vi "Facade.vi"(0 "Data In":T7={"Slider"={"Numeric"=25.0, "Numeric"=0.0, "Numeric"=0.0}, "Digital display"=0.0, "end_timer"=TRUE} {"Slider" scale=0.0..500.0 scale format="%#_5g"}, 2 "Display State In":T3={"SP_Source"={"connect"=FALSE, "SP_Source"=enum."initialize", "SP_Set"=0.0, "SP"=0.0}, "Write"=FALSE, "button state"=enum."init", "reset_timer"=FALSE, "load_timer"=FALSE, "Time"=0, "t ms"=0, "tick"=0, "scale maximum"=100.0}, 3 "Container State":T6) -> (6 "Data Out":T7={"Slider"={"Numeric"=25.0, "Numeric"=0.0, "Numeric"=0.0}, "Digital display"=0.0, "end_timer"=TRUE} {"Slider" scale=0.0..500.0 scale format="%#_5g"}, 7 "Display State Out":T3={"SP_Source"={"connect"=FALSE, "SP_Source"=enum."initialize", "SP_Set"=0.0, "SP"=0.0}, "Write"=FALSE, "button state"=enum."init", "reset_timer"=FALSE, "load_timer"=FALSE, "Time"=0, "t ms"=0, "tick"=0, "scale maximum"=100.0}, 8 "Action":T2)   [LabVIEW 2019, in "control.lvlib" / "SP_h1.xctl"]
uses:
  SP_h1.xctl
  Data.ctl
  <vilib>/_xctls/Container State.ctl
  State.ctl
  Heating/ctl/Y_source.ctl
  Y_controlState.ctl
  <vilib>/_xctls/Action.ctl
  <vilib>/_xctls/XControlSupport.lvlib
  Timer Delay/Timers.lvlib
  Heating/Heating.lvlib
panel:
  in  "setpoint":dbl step=1.0 format="%#.1f"
  in  "slider":T1(slide) scale=0.0..1000.0 scale format="%#.0f"
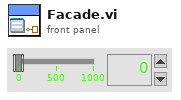
[diagram p1: front panel]
types:
  T1 = cluster{"Numeric":dbl, "Numeric":dbl, "Numeric":dbl}
  T2 = typedef "XControlSupport.lvlib/Action.ctl" = cluster{"Data Changed?":bool, "State Changed?":bool, "Action Name":string}
  T3 = typedef "control.lvlib/SP_h1.xctl/State.ctl" = cluster{"SP_Source":cluster{"connect":bool, "SP_Source":T4, "SP_Set":dbl, "SP":dbl}, "Write":bool, "button state":T5, "reset_timer":bool, "load_timer":bool, "Time":u32, "t ms":u32, "tick":u32, "scale maximum":dbl}
  T4 = typedef "Heating.lvlib/Y_source.ctl" = enum8{"initialize", "local disabled", "local hand", "hand", "auto", "dist"}
  T5 = typedef "control.lvlib/SP_h1.xctl/Y_controlState.ctl" = enum16{"init", "not connect", "local disabled", "local hand", "hand", "value change", "auto", "dist"}
  T6 = typedef "XControlSupport.lvlib/Container State.ctl" = cluster{"Indicator?":bool, "Run Mode?":bool, " Refnum":refnum<vi>}
  T7 = typedef "control.lvlib/SP_h1.xctl/Data.ctl" = cluster{"Slider":cluster{"Numeric":dbl, "Numeric":dbl, "Numeric":dbl}, "Digital display":dbl, "end_timer":bool}
  T8 = enum8{"Enabled", "Disabled", "Disabled and Grayed Out"}
  T9 = cluster{"Numeric":dbl, "NewVal":dbl, "Numeric":dbl}
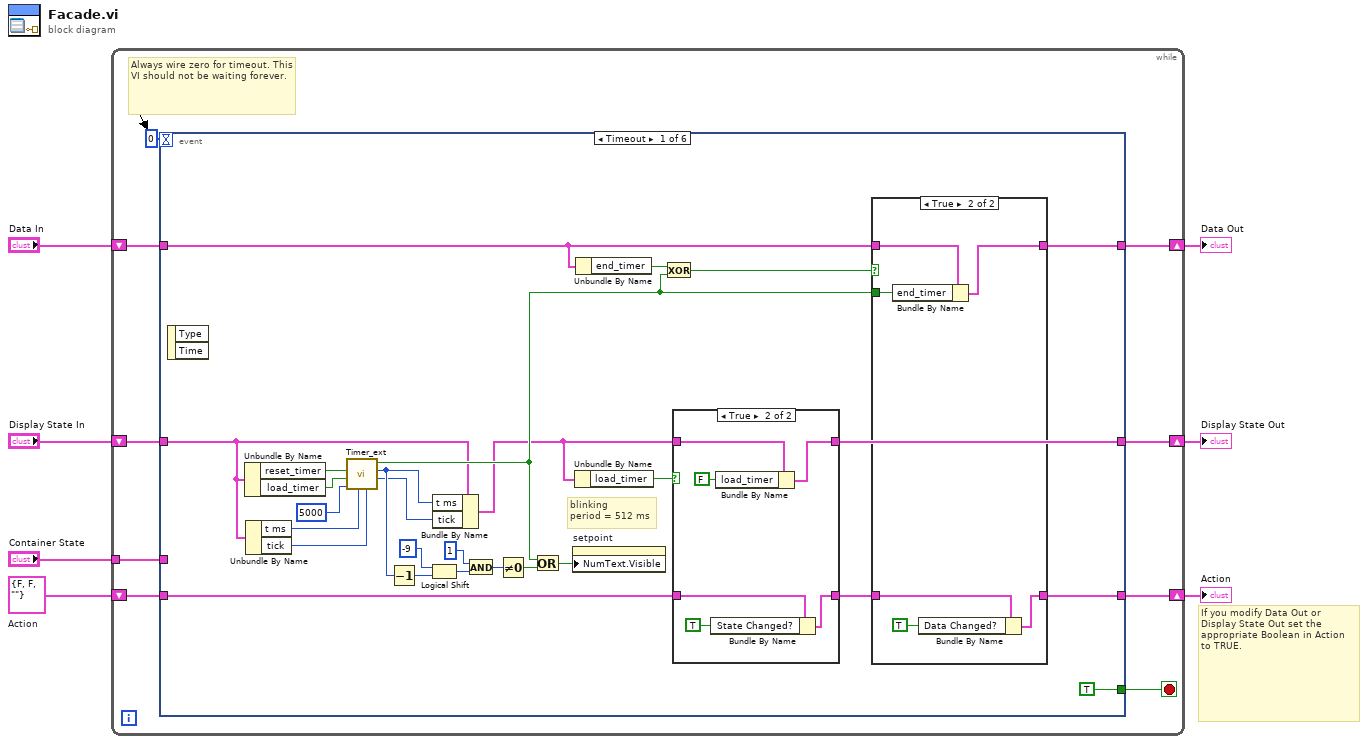
[diagram p0: block diagram]
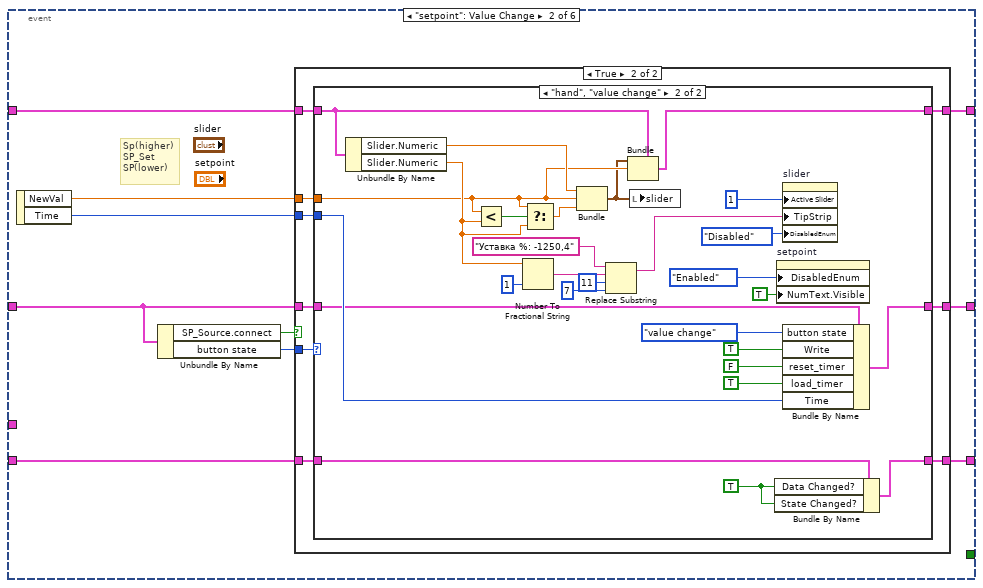
[diagram p4: hidden frame]
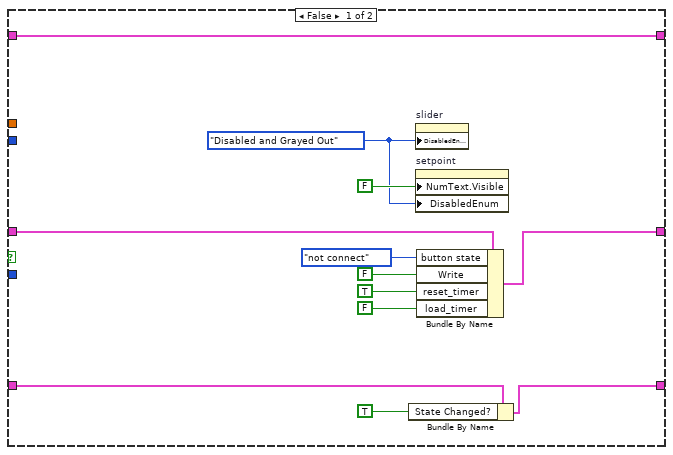
[diagram p5: hidden frame]
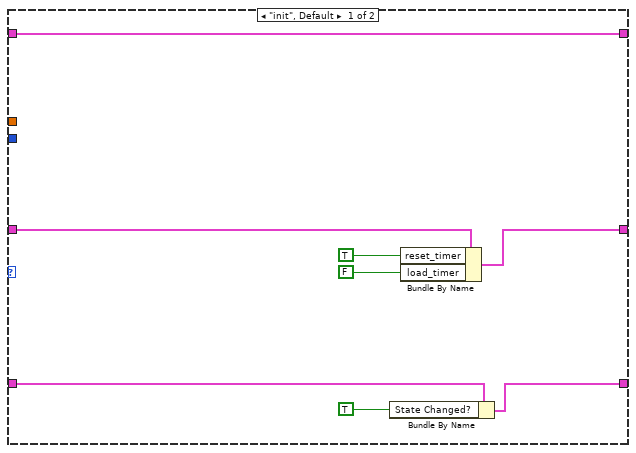
[diagram p6: hidden frame]
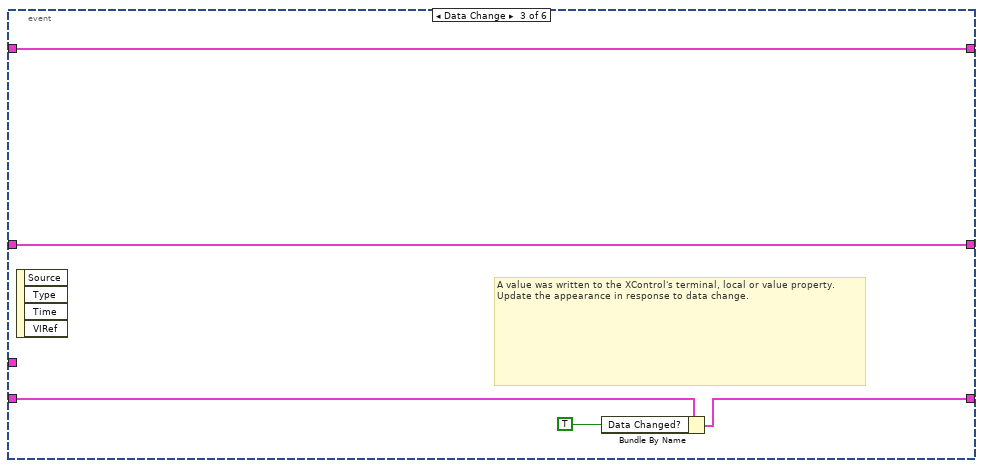
[diagram p7: hidden frame]
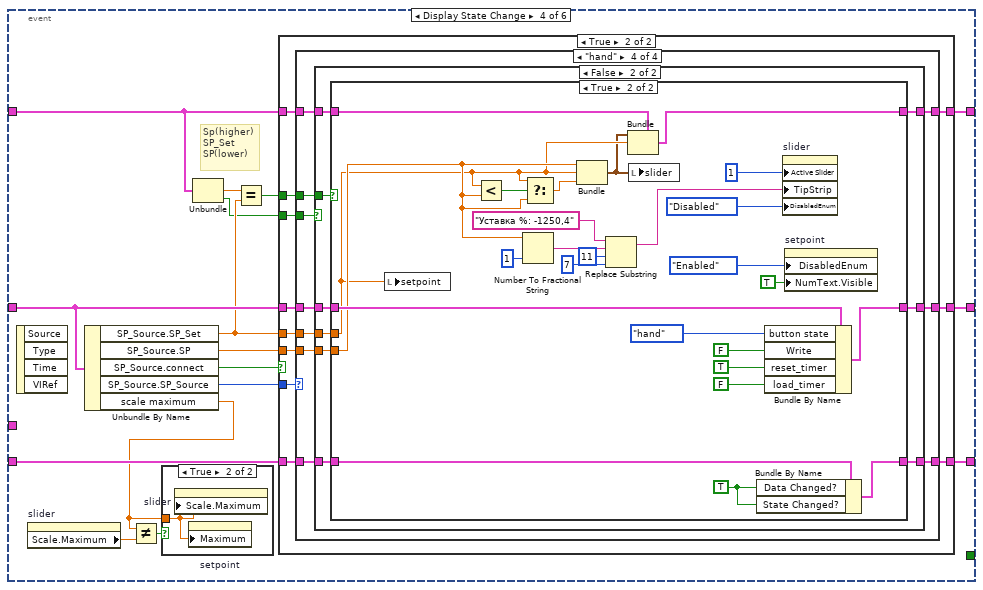
[diagram p8: hidden frame]
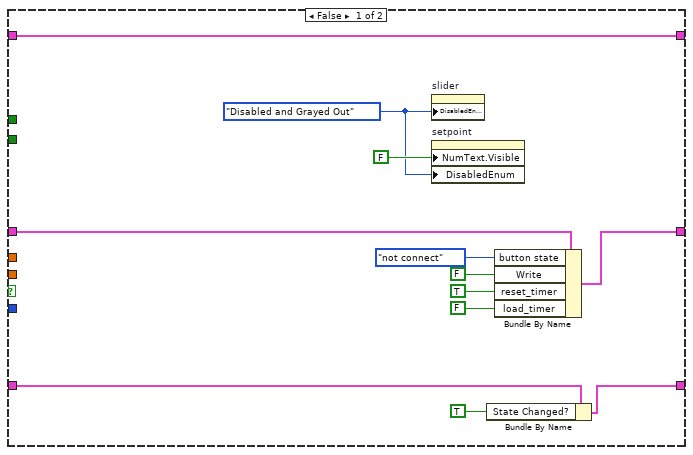
[diagram p10: hidden frame]
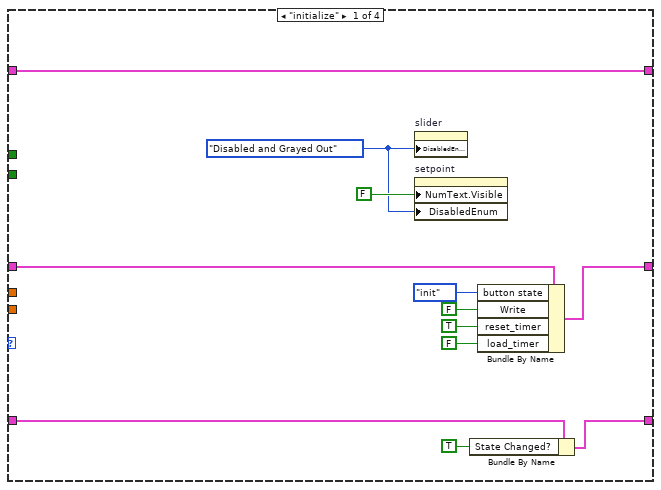
[diagram p11: hidden frame]
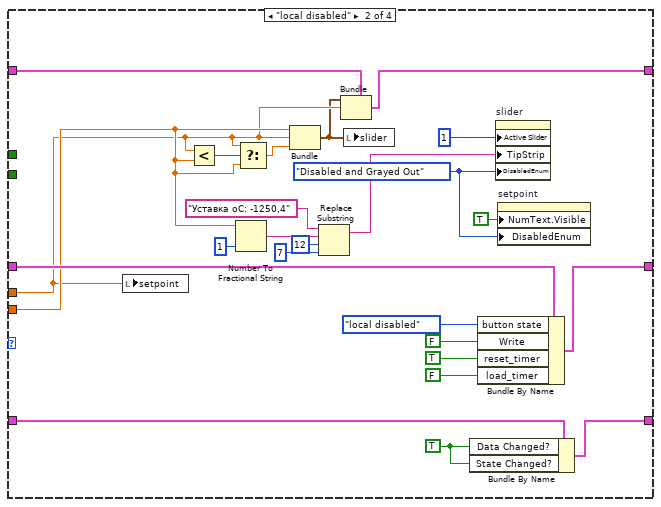
[diagram p12: hidden frame]
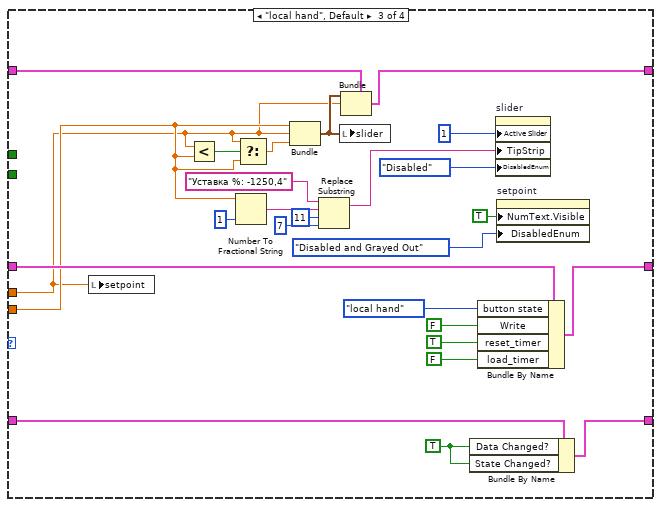
[diagram p13: hidden frame]
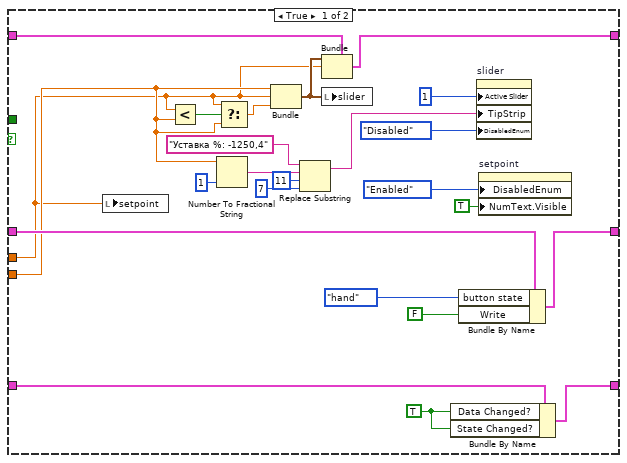
[diagram p14: hidden frame]
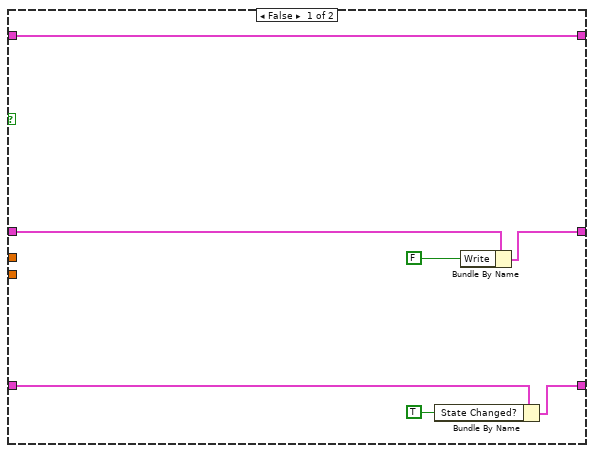
[diagram p15: hidden frame]
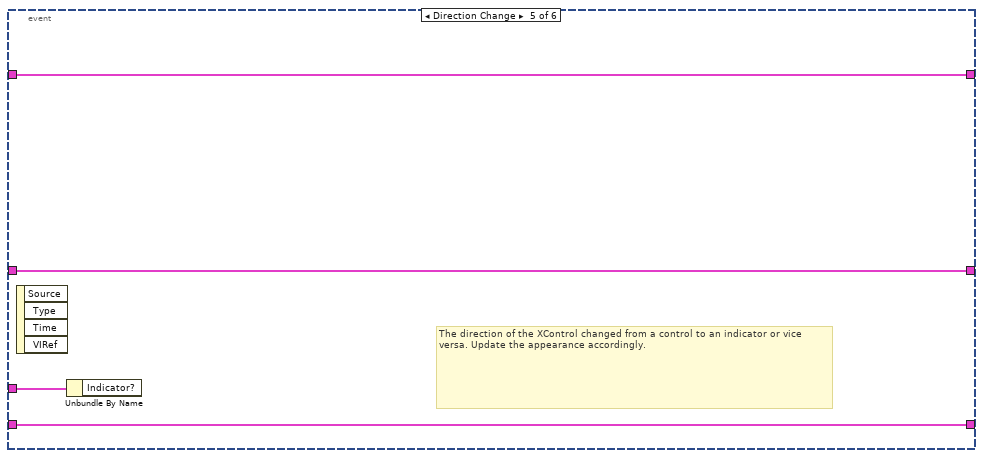
[diagram p16: hidden frame]
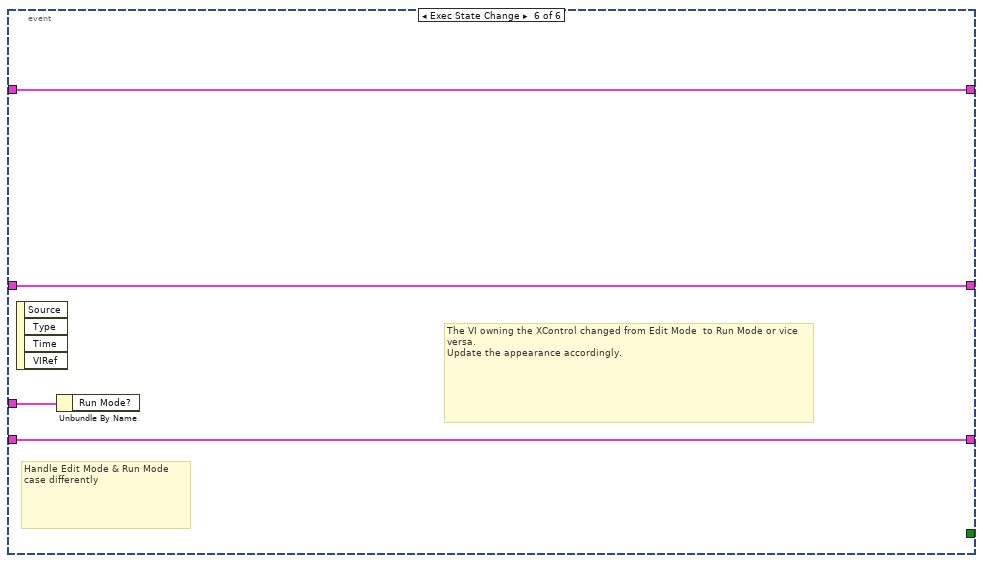
[diagram p17: hidden frame]
diagram:
  w1 = T2 {"Data Changed?"=FALSE, "State Changed?"=FALSE, "Action Name"=""}  # Action
  # "If you modify Data Out or\nDisplay State Out set the\nappropriate Boolean in Action\nto TRUE."
  n1 = while {
    shift-right: [w9] -> w4
    shift-left: "Display State In" -> [w16]
    tunnel: "Container State" -> [w13]
    shift-right: [w8] -> w7
    shift-left: "Data In" -> [w12]
    shift-right: [w10] -> w2
    shift-left: w1 -> [w11]
    stop <- w15 stop-if-true
    # "Always wire zero for timeout. This\nVI should not be waiting forever."
    n2 = event shown="[0] Timeout" {
      selector: _ -> [_ _ _ _ _ _]
      dyn-events: _ -> [_ _ _ _ _ _]
      timeout: 0 -> [_ _ _ _ _ _]
      tunnel: w16 -> [w17 w64 w130 w142 w313 w317]
      tunnel: [w40 w69 w130 w146 w313 w317] -> w9
      tunnel: [TRUE _ _ _ _ _] -> w15
      tunnel: w13 -> [_ _ _ _ w314 w318]
      tunnel: w12 -> [w28 w68 w131 w138 w312 w316]
      tunnel: [w31 w67 w131 w147 w312 w316] -> w8
      tunnel: [w23 w65 w128 w144 w311 w315] -> w10
      tunnel: w11 -> [w29 w66 w127 w145 w311 w315]
      event Timeout {
        # "blinking\nperiod = 512 ms"
        n3 = event-data() -> ()  [unwired: 1 in, 2 out]
        n4 = Unbundle By Name(w17) -> ("reset_timer"=w42:bool, "load_timer"=w41:bool)
        n5 = Unbundle By Name(w17) -> ("t ms"=w22:u32, "tick"=w21:u32)
        n6 = call "Timer_ext.vi"("tick old"=w21, "t ms old"=w22, "ms"=u32 5000, "Load"=w41, "Reset"=w42) -> ("tick"=w19:u32, "t ms"=w20:u32, "End"=w26:bool)  [unwired: 4 in]
        n7 = Decrement(x=w20) -> (x-1=w37:u32)
        n8 = Logical Shift(y=i16 -9, x=w37) -> (x << y=w35:u32)
        n9 = Bundle By Name(cluster=w17, "t ms"=w20, "tick"=w19) -> (w18:T3)
        n10 = And(x=u32 1 ("y"), y=w35) -> (x .and. y?=w33:u32)
        n11 = Not Equal To 0?(x=w33) -> (x != 0?=w38:bool)
        n12 = Or(x=w26, y=w38) -> (x .or. y?=w32:bool)
        n13 = property on="setpoint" class="DigNum (strict)"("NumText.Visible"=w32) -> ()  [unwired: 2 in, 2 out]
        n14 = Unbundle By Name(w18) -> ("load_timer"=w30:bool)
        n15 = Unbundle By Name(w28) -> ("end_timer"=w27:bool)
        n16 = Exclusive Or(1:w26, 2:w27) -> (0:w25:bool)
        n17 = case shown="True" w30 {
          tunnel: [w53 w59] -> w40
          tunnel: w18 -> [w53 w57]
          tunnel: w29 -> [w52 w55]
          tunnel: [w52 w54] -> w24
          frame False {
          }
          frame True {
            n18 = Bundle By Name(cluster=w55, "State Changed?"=TRUE ("Data Changed?")) -> (w54:T2)
            n19 = Bundle By Name(cluster=w57, "load_timer"=FALSE) -> (w59:T3)
          }
        }
        n20 = case shown="True" w25 {
          tunnel: [w44 w51] -> w31
          tunnel: w28 -> [w44 w50]
          tunnel: w26 -> [_ w49]
          tunnel: w24 -> [w45 w47]
          tunnel: [w45 w46] -> w23
          frame False {
          }
          frame True {
            n21 = Bundle By Name(cluster=w50, "end_timer"=w49) -> (w51:T7)
            n22 = Bundle By Name(cluster=w47, "Data Changed?"=TRUE) -> (w46:T2)
          }
        }
      }
      event "setpoint": Value Change {
        # "Sp(higher)\nSP_Set\nSP(lower)"
        n23 = event-data() -> ("NewVal"=w61:dbl, "Time"=w60:u32)  [unwired: 1 in]
        n24 = Unbundle By Name(w64) -> ("SP_Source.connect"=w63:bool, "button state"=w62:T5)
        n25 = case shown="True" w63 {
          tunnel: w62 -> [_ w90]
          tunnel: w64 -> [w80 w89]
          tunnel: [w79 w88] -> w69
          tunnel: w68 -> [w72 w87]
          tunnel: [w72 w86] -> w67
          tunnel: w66 -> [w77 w84]
          tunnel: [w76 w85] -> w65
          tunnel: w61 -> [_ w83]
          tunnel: w60 -> [_ w82]
          frame False {
            w70 = T8."Disabled and Grayed Out" ("Disabled")
            n26 = Bundle By Name(cluster=w77, "State Changed?"=TRUE ("Data Changed?")) -> (w76:T2)
            n27 = property on="slider" class="Slide (strict)"("DisabledEnum"=w70) -> ()  [unwired: 2 in, 2 out]
            n28 = property on="setpoint" class="DigNum (strict)"("NumText.Visible"=FALSE ("Z_ASwitch"), "DisabledEnum"=w70) -> ()  [unwired: 2 in, 2 out]
            n29 = Bundle By Name(cluster=w80, "button state"=Y_controlState."not connect" ("f 3"), "Write"=FALSE ("Z_ASwitch"), "reset_timer"=TRUE ("Z_ASwitch"), "load_timer"=FALSE ("Z_ASwitch")) -> (w79:T3)
          }
          frame True {
            n30 = case shown="\"hand\", \"value change\"" w90 {
              tunnel: w89 -> [w97 w108]
              tunnel: [w96 w126] -> w88
              tunnel: w87 -> [w91 w105]
              tunnel: [w91 w107] -> w86
              tunnel: [w93 w124] -> w85
              tunnel: w84 -> [w94 w125]
              tunnel: w83 -> [_ w102]
              tunnel: w82 -> [_ w109]
              frame "init", Default {
                # "local hand"
                n31 = Bundle By Name(cluster=w94, "State Changed?"=TRUE ("Data Changed?")) -> (w93:T2)
                n32 = Bundle By Name(cluster=w97, "reset_timer"=TRUE, "load_timer"=FALSE) -> (w96:T3)
              }
              frame "hand", "value change" {
                w120 = TRUE ("Data Changed?")
                # "local hand"
                n33 = Unbundle By Name(w105) -> ("Slider.Numeric"=w104:dbl, "Slider.Numeric"=w103:dbl)
                n34 = Less?(x=w102, y=w103) -> (x < y?=w113:bool)
                n35 = Number To Fractional String(number=w103, precision (6)=i16 1) -> (F-format string=w116:string)  [unwired: 2 in]
                n36 = Select(t=w102, s=w113, f=w103) -> (s? t:f=w112:dbl)
                n37 = Bundle("Numeric"=w104, "NewVal"=w102, "Numeric"=w112) -> (w99:T9)  [unwired: 1 in]
                n38 = Replace Substring(2:7 ("length (len. of substring)"), 3:11 ("offset (0)"), 4:w116, 5:"Уставка %: -1250,4") -> (1:w110:string)  [unwired: 1 out]
                n39 = Bundle(cluster=w105, "Slider"=w99, "Digital display"=w102) -> (w107:T7)  [unwired: 1 in]
                n40 = local write "slider"(w99) -> ()
                n41 = Bundle By Name(cluster=w125, "Data Changed?"=w120, "State Changed?"=w120) -> (w124:T2)
                n42 = property on="setpoint" class="DigNum (strict)"("DisabledEnum"=T8."Enabled" ("Disabled"), "NumText.Visible"=TRUE ("Numeric Text.Visible")) -> ()  [unwired: 2 in, 2 out]
                n43 = property on="slider" class="Slide (strict)"("Active Slider"=1, "TipStrip"=w110, "DisabledEnum"=T8."Disabled" ("Disabled")) -> ()  [unwired: 2 in, 2 out]
                n44 = Bundle By Name(cluster=w108, "button state"=Y_controlState."value change" ("f 3"), "Write"=TRUE ("Z_ASwitch"), "reset_timer"=FALSE ("Z_ASwitch"), "load_timer"=TRUE ("Z_ASwitch"), "Time"=w109) -> (w126:T3)
              }
            }
          }
        }
      }
      event Data Change {
        # "A value was written to the XControl's terminal, local or value property.\nUpdate the appearance in response to data change."
        n45 = event-data() -> ()  [unwired: 1 in, 4 out]
        n46 = Bundle By Name(cluster=w127, "Data Changed?"=TRUE) -> (w128:T2)
      }
      event Display State Change {
        # "Sp(higher)\nSP_Set\nSP(lower)"
        n47 = event-data() -> ()  [unwired: 1 in, 4 out]
        n48 = property on="slider" class="Slide (strict)"() -> ("Scale.Maximum"=w135:dbl)  [unwired: 2 in, 2 out]
        n49 = Unbundle By Name(w142) -> ("SP_Source.SP_Set"=w136:dbl, "SP_Source.SP"=w139:dbl, "SP_Source.connect"=w143:bool, "SP_Source.SP_Source"=w141:T4, "scale maximum"=w134:dbl)
        n50 = Not Equal?(x=w134, y=w135) -> (x != y?=w133:bool)
        n51 = case shown="True" w133 {
          tunnel: w134 -> [_ w148]
          frame False {
          }
          frame True {
            n52 = property on="slider" class="Slide (strict)"("Scale.Maximum"=w148) -> ()  [unwired: 2 in, 2 out]
            n53 = property on="setpoint" class="DigNum (strict)"("Maximum"=w148) -> ()  [unwired: 2 in, 2 out]
          }
        }
        n54 = Unbundle(w138) -> ("Digital display"=w137:dbl, "end_timer"=w132:bool)  [unwired: 1 out]
        n55 = Equal?(x=w137, y=w136) -> (x = y?=w140:bool)
        n56 = case shown="True" w143 {
          tunnel: w141 -> [_ w171]
          tunnel: w142 -> [w159 w170]
          tunnel: [w158 w169] -> w146
          tunnel: w138 -> [w151 w168]
          tunnel: [w151 w167] -> w147
          tunnel: w145 -> [w156 w165]
          tunnel: [w155 w166] -> w144
          tunnel: w132 -> [_ w164]
          tunnel: w139 -> [_ w163]
          tunnel: w140 -> [_ w162]
          tunnel: w136 -> [_ w161]
          frame False {
            w149 = T8."Disabled and Grayed Out" ("Disabled")
            n57 = property on="slider" class="Slide (strict)"("DisabledEnum"=w149) -> ()  [unwired: 2 in, 2 out]
            n58 = property on="setpoint" class="DigNum (strict)"("NumText.Visible"=FALSE ("Z_ASwitch"), "DisabledEnum"=w149) -> ()  [unwired: 2 in, 2 out]
            n59 = Bundle By Name(cluster=w156, "State Changed?"=TRUE ("Data Changed?")) -> (w155:T2)
            n60 = Bundle By Name(cluster=w159, "button state"=Y_controlState."not connect" ("f 3"), "Write"=FALSE ("Z_ASwitch"), "reset_timer"=TRUE ("Z_ASwitch"), "load_timer"=FALSE ("Z_ASwitch")) -> (w158:T3)
          }
          frame True {
            n61 = case shown="\"hand\"" w171 {
              tunnel: w170 -> [w183 w208 w234 w244]
              tunnel: [w182 w207 w233 w243] -> w169
              tunnel: w168 -> [w174 w189 w214 w237]
              tunnel: [w174 w190 w215 w238] -> w167
              tunnel: [w180 w205 w231 w241] -> w166
              tunnel: w165 -> [w181 w206 w232 w242]
              tunnel: w164 -> [_ _ _ w240]
              tunnel: w163 -> [_ w188 w212 w239]
              tunnel: w162 -> [_ _ _ w236]
              tunnel: w161 -> [_ w185 w209 w235]
              frame "initialize" {
                w172 = T8."Disabled and Grayed Out" ("Disabled")
                # "local hand"
                n62 = property on="slider" class="Slide (strict)"("DisabledEnum"=w172) -> ()  [unwired: 2 in, 2 out]
                n63 = property on="setpoint" class="DigNum (strict)"("NumText.Visible"=FALSE ("Z_ASwitch"), "DisabledEnum"=w172) -> ()  [unwired: 2 in, 2 out]
                n64 = Bundle By Name(cluster=w181, "State Changed?"=TRUE ("Data Changed?")) -> (w180:T2)
                n65 = Bundle By Name(cluster=w183, "button state"=Y_controlState."init" ("f 3"), "Write"=FALSE ("Z_ASwitch"), "reset_timer"=TRUE ("Z_ASwitch"), "load_timer"=FALSE ("Z_ASwitch")) -> (w182:T3)
              }
              frame "local disabled" {
                w186 = T8."Disabled and Grayed Out" ("Disabled")
                w200 = TRUE ("Data Changed?")
                # "local hand"
                n66 = local write "setpoint"(w185) -> ()
                n67 = Less?(x=w185, y=w188) -> (x < y?=w194:bool)
                n68 = Number To Fractional String(number=w188, precision (6)=i16 1) -> (F-format string=w197:string)  [unwired: 2 in]
                n69 = Select(t=w185, s=w194, f=w188) -> (s? t:f=w193:dbl)
                n70 = Bundle("SP"=w188, "SP_Set"=w185, "SP"=w193) -> (w184:cluster{"SP":dbl, "SP_Set":dbl, "SP":dbl})  [unwired: 1 in]
                n71 = Replace Substring(2:7 ("length (len. of substring)"), 3:12 ("offset (0)"), 4:w197, 5:"Уставка оС: -1250,4") -> (1:w191:string)  [unwired: 1 out]
                n72 = Bundle(cluster=w189, "Slider"=w184, "Digital display"=w185) -> (w190:T7)  [unwired: 1 in]
                n73 = local write "slider"(w184) -> ()
                n74 = Bundle By Name(cluster=w206, "Data Changed?"=w200, "State Changed?"=w200) -> (w205:T2)
                n75 = Bundle By Name(cluster=w208, "button state"=Y_controlState."local disabled" ("f 3"), "Write"=FALSE ("Z_ASwitch"), "reset_timer"=TRUE ("Z_ASwitch"), "load_timer"=FALSE ("Z_ASwitch")) -> (w207:T3)
                n76 = property on="slider" class="Slide (strict)"("Active Slider"=1, "TipStrip"=w191, "DisabledEnum"=w186) -> ()  [unwired: 2 in, 2 out]
                n77 = property on="setpoint" class="DigNum (strict)"("NumText.Visible"=TRUE ("Numeric Text.Visible"), "DisabledEnum"=w186) -> ()  [unwired: 2 in, 2 out]
              }
              frame "local hand", Default {
                w226 = TRUE ("Data Changed?")
                # "local hand"
                n78 = local write "setpoint"(w209) -> ()
                n79 = Less?(x=w209, y=w212) -> (x < y?=w220:bool)
                n80 = Number To Fractional String(number=w212, precision (6)=i16 1) -> (F-format string=w223:string)  [unwired: 2 in]
                n81 = Select(t=w209, s=w220, f=w212) -> (s? t:f=w219:dbl)
                n82 = Bundle("SP"=w212, "SP_Set"=w209, "SP"=w219) -> (w210:cluster{"SP":dbl, "SP_Set":dbl, "SP":dbl})  [unwired: 1 in]
                n83 = Replace Substring(2:7 ("length (len. of substring)"), 3:11 ("offset (0)"), 4:w223, 5:"Уставка %: -1250,4") -> (1:w217:string)  [unwired: 1 out]
                n84 = local write "slider"(w210) -> ()
                n85 = Bundle(cluster=w214, "Slider"=w210, "Digital display"=w209) -> (w215:T7)  [unwired: 1 in]
                n86 = Bundle By Name(cluster=w232, "Data Changed?"=w226, "State Changed?"=w226) -> (w231:T2)
                n87 = Bundle By Name(cluster=w234, "button state"=Y_controlState."local hand" ("f 3"), "Write"=FALSE ("Z_ASwitch"), "reset_timer"=TRUE ("Z_ASwitch"), "load_timer"=FALSE ("Z_ASwitch")) -> (w233:T3)
                n88 = property on="slider" class="Slide (strict)"("Active Slider"=1, "TipStrip"=w217, "DisabledEnum"=T8."Disabled" ("Disabled")) -> ()  [unwired: 2 in, 2 out]
                n89 = property on="setpoint" class="DigNum (strict)"("NumText.Visible"=TRUE ("Numeric Text.Visible"), "DisabledEnum"=T8."Disabled and Grayed Out" ("Disabled")) -> ()  [unwired: 2 in, 2 out]
              }
              frame "hand" {
                # "local hand"
                n90 = case shown="False" w240 {
                  tunnel: w244 -> [w268 w277]
                  tunnel: [w267 w276] -> w243
                  tunnel: w242 -> [w266 w275]
                  tunnel: [w265 w274] -> w241
                  tunnel: w239 -> [w250 w271]
                  tunnel: [w252 w273] -> w238
                  tunnel: w237 -> [w251 w272]
                  tunnel: w236 -> [_ w270]
                  tunnel: w235 -> [w245 w269]
                  frame True {
                    w262 = TRUE ("Data Changed?")
                    n91 = local write "setpoint"(w245) -> ()
                    n92 = Less?(x=w245, y=w250) -> (x < y?=w256:bool)
                    n93 = Number To Fractional String(number=w250, precision (6)=i16 1) -> (F-format string=w259:string)  [unwired: 2 in]
                    n94 = Select(t=w245, s=w256, f=w250) -> (s? t:f=w255:dbl)
                    n95 = Bundle("SP"=w250, "SP_Set"=w245, "SP"=w255) -> (w246:cluster{"SP":dbl, "SP_Set":dbl, "SP":dbl})  [unwired: 1 in]
                    n96 = Replace Substring(2:7 ("length (len. of substring)"), 3:11 ("offset (0)"), 4:w259, 5:"Уставка %: -1250,4") -> (1:w253:string)  [unwired: 1 out]
                    n97 = Bundle(cluster=w251, "Slider"=w246, "Digital display"=w245) -> (w252:T7)  [unwired: 1 in]
                    n98 = local write "slider"(w246) -> ()
                    n99 = Bundle By Name(cluster=w266, "Data Changed?"=w262, "State Changed?"=w262) -> (w265:T2)
                    n100 = Bundle By Name(cluster=w268, "button state"=Y_controlState."hand" ("f 3"), "Write"=FALSE ("Z_ASwitch")) -> (w267:T3)
                    n101 = property on="slider" class="Slide (strict)"("Active Slider"=1, "TipStrip"=w253, "DisabledEnum"=T8."Disabled" ("Disabled")) -> ()  [unwired: 2 in, 2 out]
                    n102 = property on="setpoint" class="DigNum (strict)"("DisabledEnum"=T8."Enabled" ("Disabled"), "NumText.Visible"=TRUE ("Numeric Text.Visible")) -> ()  [unwired: 2 in, 2 out]
                  }
                  frame False {
                    n103 = case shown="True" w270 {
                      tunnel: w277 -> [w280 w310]
                      tunnel: [w279 w309] -> w276
                      tunnel: w275 -> [w283 w308]
                      tunnel: [w281 w307] -> w274
                      tunnel: [w284 w289] -> w273
                      tunnel: w272 -> [w284 w290]
                      tunnel: w271 -> [_ w288]
                      tunnel: w269 -> [_ w286]
                      frame False {
                        n104 = Bundle By Name(cluster=w283, "State Changed?"=TRUE ("Data Changed?")) -> (w281:T2)
                        n105 = Bundle By Name(cluster=w280, "Write"=FALSE ("Z_ASwitch")) -> (w279:T3)
                      }
                      frame True {
                        w304 = TRUE ("Data Changed?")
                        n106 = local write "setpoint"(w286) -> ()
                        n107 = Less?(x=w286, y=w288) -> (x < y?=w296:bool)
                        n108 = Number To Fractional String(number=w288, precision (6)=i16 1) -> (F-format string=w299:string)  [unwired: 2 in]
                        n109 = Select(t=w286, s=w296, f=w288) -> (s? t:f=w295:dbl)
                        n110 = Bundle("SP"=w288, "SP_Set"=w286, "SP"=w295) -> (w285:cluster{"SP":dbl, "SP_Set":dbl, "SP":dbl})  [unwired: 1 in]
                        n111 = Replace Substring(2:7 ("length (len. of substring)"), 3:11 ("offset (0)"), 4:w299, 5:"Уставка %: -1250,4") -> (1:w293:string)  [unwired: 1 out]
                        n112 = Bundle(cluster=w290, "Slider"=w285, "Digital display"=w286) -> (w289:T7)  [unwired: 1 in]
                        n113 = local write "slider"(w285) -> ()
                        n114 = Bundle By Name(cluster=w308, "Data Changed?"=w304, "State Changed?"=w304) -> (w307:T2)
                        n115 = Bundle By Name(cluster=w310, "button state"=Y_controlState."hand" ("f 3"), "Write"=FALSE ("Z_ASwitch"), "reset_timer"=TRUE ("Z_ASwitch"), "load_timer"=FALSE ("Z_ASwitch")) -> (w309:T3)
                        n116 = property on="slider" class="Slide (strict)"("Active Slider"=1, "TipStrip"=w293, "DisabledEnum"=T8."Disabled" ("Disabled")) -> ()  [unwired: 2 in, 2 out]
                        n117 = property on="setpoint" class="DigNum (strict)"("DisabledEnum"=T8."Enabled" ("Disabled"), "NumText.Visible"=TRUE ("Numeric Text.Visible")) -> ()  [unwired: 2 in, 2 out]
                      }
                    }
                  }
                }
              }
            }
          }
        }
      }
      event Direction Change {
        # "The direction of the XControl changed from a control to an indicator or vice versa. Update the appearance accordingly."
        n118 = event-data() -> ()  [unwired: 1 in, 4 out]
        n119 = Unbundle By Name(w314) -> ()  [unwired: 1 out]
      }
      event Exec State Change {
        # "The VI owning the XControl changed from Edit Mode  to Run Mode or vice versa.\nUpdate the appearance accordingly."
        # "Handle Edit Mode & Run Mode\ncase differently"
        n120 = event-data() -> ()  [unwired: 1 in, 4 out]
        n121 = Unbundle By Name(w318) -> ()  [unwired: 1 out]
      }
    }
  }
  "Display State Out" <- w4
  "Data Out" <- w7
  "Action" <- w2
